vi "test Get and Set All.vi"(8 "error in (no error)":errorcluster, 11 "TestCase in":refnum<class "Variant Data Manipulation Tests.lvclass">) -> (0 "error out":errorcluster, 3 "TestCase out":refnum<class "Variant Data Manipulation Tests.lvclass">)   [LabVIEW 2017, in "Variant Data Manipulation Tests.lvclass"]
uses:
  Variant Data Manipulation Tests.lvclass
  <vilib>/addons/_JKI Toolkits/VI Tester/TestCase.llb/TestCase.lvclass
  Source/Variant Data Manipulation.lvlib
  <vilib>/Utility/Data Type/NI_Data Type.lvlib
  C:/Program Files (x86)/National Instruments/LabVIEW 2017/vi.lib/addons/_JKI Toolkits/VI Tester/TestCase.llb/TestCase.lvclass
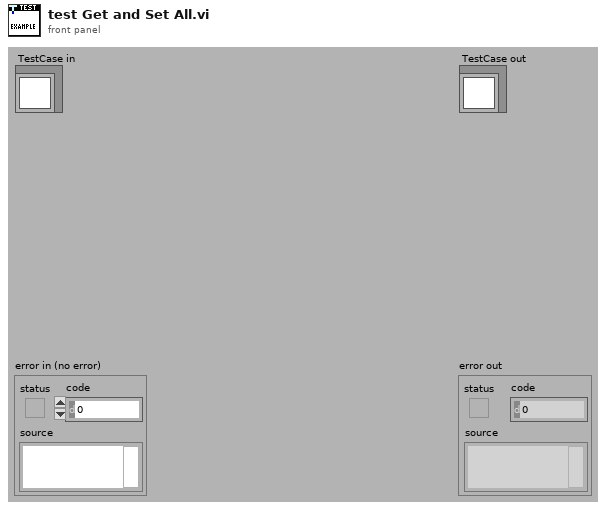
[diagram p1: front panel]
types:
  T1 = cluster{"String":string, "Boolean":bool, "Numeric":dbl}
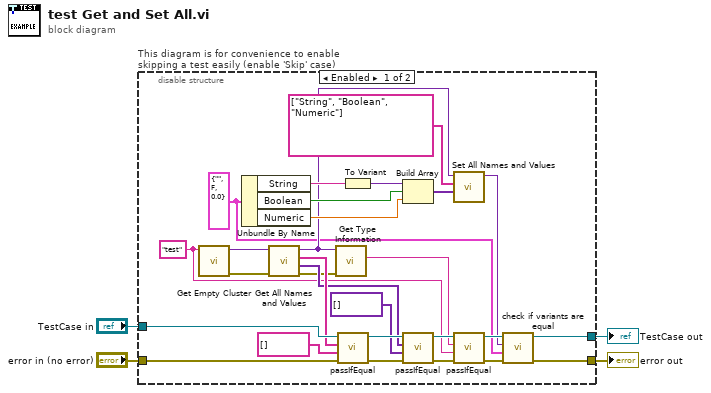
[diagram p0: block diagram]
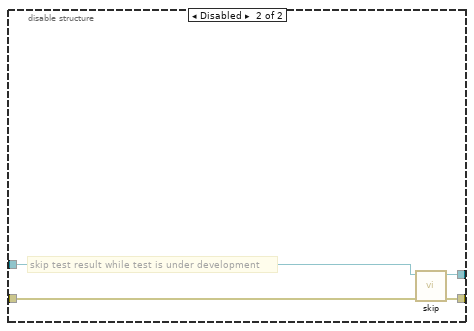
[diagram p2: hidden frame]
diagram:
  n1 = disable-structure "This diagram is for convenience to enable skipping a test easily (enable 'Skip' case)" shown="Enabled" {
    disable-tunnel: "TestCase in" -> [w32 w36]
    disable-tunnel: [w5 w34] -> w1
    disable-tunnel: [w6 w35] -> w3
    disable-tunnel: "error in (no error)" -> [w30 w33]
    frame Enabled {
      w8 = T1 {"String"="", "Boolean"=FALSE, "Numeric"=0.0} ("Cluster")
      w19 = "test" ("Name")
      n2 = call "Get Empty Cluster.vi"("Name"=w19) -> ("error out"=w28:errorcluster, "Variant (Cluster) out"=w29:variant)  [unwired: 9 in]
      n3 = Unbundle By Name(w8) -> ("String"=w17:string, "Boolean"=w16:bool, "Numeric"=w15:dbl)
      n4 = call "Get All Names and Values.vi"("error in"=w28, "Cluster in"=w29) -> ("error out"=w18:errorcluster, "Values"=w24:variant[], "Element Names"=w25:string[], "Cluster out"=w13:variant)  [unwired: 5 in, 1 out]
      n5 = call <vilib>:"Get Type Information.vi"("error in (no error)"=w18, "Variant"=w13) -> ("Name"=w20:string)  [unwired: 5 in, 4 out]
      n6 = call-dynamic "passIfEqual.vi"("error in (no error)"=w30, "y"=string[] [] ("Element Names"), "x"=w25, "TestCase in"=w32) -> ("error out"=w31:errorcluster, "TestCase out"=w26:refnum<class "Variant Data Manipulation Tests.lvclass">)  [unwired: 6 in]
      n7 = To Variant(anything=w17) -> (Variant=w14:variant)
      n8 = Build Array(w14, w16, w15) -> (w12:variant[])
      n9 = call-dynamic "passIfEqual.vi"("error in (no error)"=w31, "y"=variant[] [] ("Values"), "x"=w24, "TestCase in"=w26) -> ("error out"=w27:errorcluster, "TestCase out"=w21:refnum<class "Variant Data Manipulation Tests.lvclass">)  [unwired: 6 in]
      n10 = call "Set All Names and Values.vi"("values"=w12, "Element Names"=string[] ["String", "Boolean", "Numeric"], "Cluster in"=w13) -> ("Cluster out"=w9:variant)  [unwired: 7 in, 1 out]
      n11 = call-dynamic "passIfEqual.vi"("error in (no error)"=w27, "y"=w19, "x"=w20, "TestCase in"=w21) -> ("error out"=w7:errorcluster, "TestCase out"=w10:refnum<class "Variant Data Manipulation Tests.lvclass">)  [unwired: 6 in]
      n12 = call "check if variants are equal.vi"("error in (no error)"=w7, 9:"Variant in"=w8, 10:"Variant in"=w9, "Dynamic Cluster Test in"=w10) -> ("error out"=w6:errorcluster, "Dynamic Cluster Test out"=w5:refnum<class "Variant Data Manipulation Tests.lvclass">)  [unwired: 6 in]
    }
    frame Disabled {
      # "skip test result while test is under development"
      n13 = call <vilib>:"skip.vi"("error in (no error)"=w33, "TestCase in"=w36) -> ("error out"=w35:errorcluster, "TestCase out"=w34:refnum<class "Variant Data Manipulation Tests.lvclass">)  [unwired: 8 in]
    }
  }
  "error out" <- w3
  "TestCase out" <- w1
